vi "Shutdown Transceiver.vi"(8 "error in (no error)":errorcluster, 11 "UDP Transceiver in":refnum<class "UDP Transceiver.lvclass">) -> (0 "error out":errorcluster, 3 "UDP Transceiver out":refnum<class "UDP Transceiver.lvclass">)   [LabVIEW 2017, in "UDP Transceiver.lvlib" / "UDP Transceiver.lvclass"]
uses:
  UDP Transceiver.lvclass
  UDP Transceiver.lvclass/UDP Transceiver.ctl
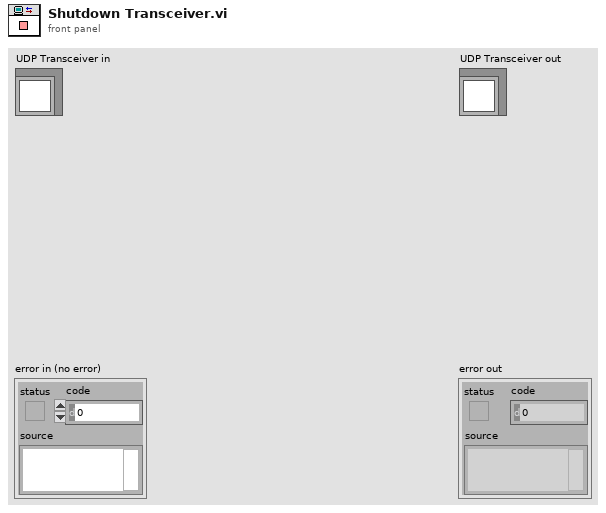
[diagram p1: front panel]
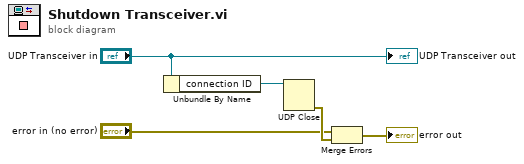
[diagram p0: block diagram]
diagram:
  n1 = Unbundle By Name("UDP Transceiver in") -> ("connection ID"=w5:refnum<k16>)
  n2 = UDP Close(connection ID=w5) -> (error out=w3:errorcluster)  [unwired: 1 in, 1 out]
  n3 = Merge Errors("error in (no error)", w3) -> (→"error out":errorcluster)
  "UDP Transceiver out" <- "UDP Transceiver in"
